vi "KlingerV2 AxisParams.vi"(0 "Axe":u8(ring) items=["W", "X", "Y", "Z"], 1 "TypeMouv":i32(ring) caption="Type de mouvement" items=["Linéaire", "Rotation"], 2 "Nom de l'axe":string, 5 "Type":i32(ring) caption="Type de moteur" items=["UE30", "UE72"], 7 "FactConv":dbl=0.01 caption="Facteur de\nConversion\n(m/pas ou °/pas)", 11 "error in":errorcluster, 12 "Encodeur":bool caption="Possède un\nEncodeur", 13 "MiseàZéro":bool caption="Possède un\nInterrupteur d'origine") -> (4 "Encodeur Out":bool caption="Possède un\nEncodeur", 6 "Nom Out":string, 8 "CorrParams out":T1={"CorrActive"=FALSE, "ErreurLim"=0.1, "NbrEssais"=3} caption="Paramètres de \ncorrection de position" {"NbrEssais" min=1 max=5 step=1; "ErreurLim" min=0.0 max=10.0 step=0.1 format="%#.1f"}, 15 "error out":errorcluster)   [LabVIEW 2019]
doc: "Ce Vi de lire et d'écrire les paramètres des différents axes du fichier .ini"
uses:
  <userlib>/KlingerV2/KlingerV2 Params.ctl
panel:
  in  "CorrParams":T1={"CorrActive"=FALSE, "ErreurLim"=0.1, "NbrEssais"=3} caption="Paramètres de \ncorrection de position" {"NbrEssais" min=1 max=5 step=1; "ErreurLim" min=0.0 max=10.0 step=0.1 format="%#.1f"}
  in  "Id Num":i32 caption="Numéro Id."
  in  "Quitter":bool
  in  "Save":bool
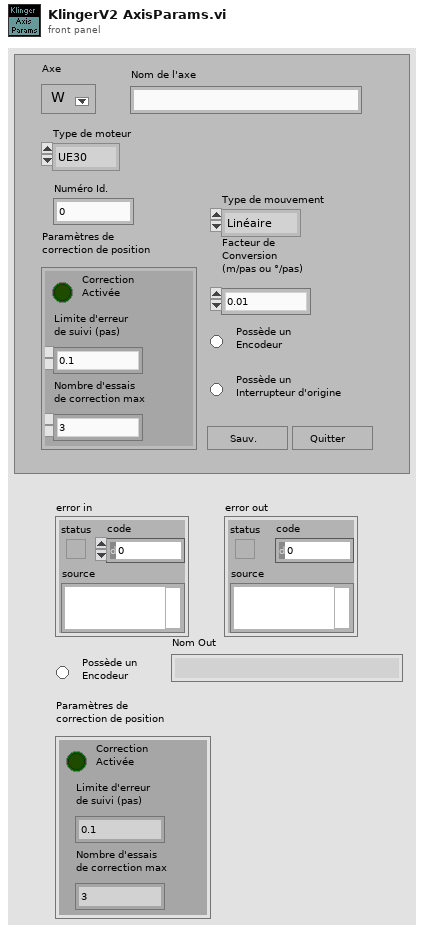
[diagram p1: front panel]
types:
  T1 = cluster{"CorrActive":bool, "ErreurLim":dbl, "NbrEssais":i32}
  T2 = typedef "KlingerV2 Params.ctl" = enum16{"Type", "Origine", "Encodeur", "TypeMouv", "FactConv", "Nom", "CorrParams", "KlingCtrlPar", "Speed", "Acc", "Avance", "Tous"}
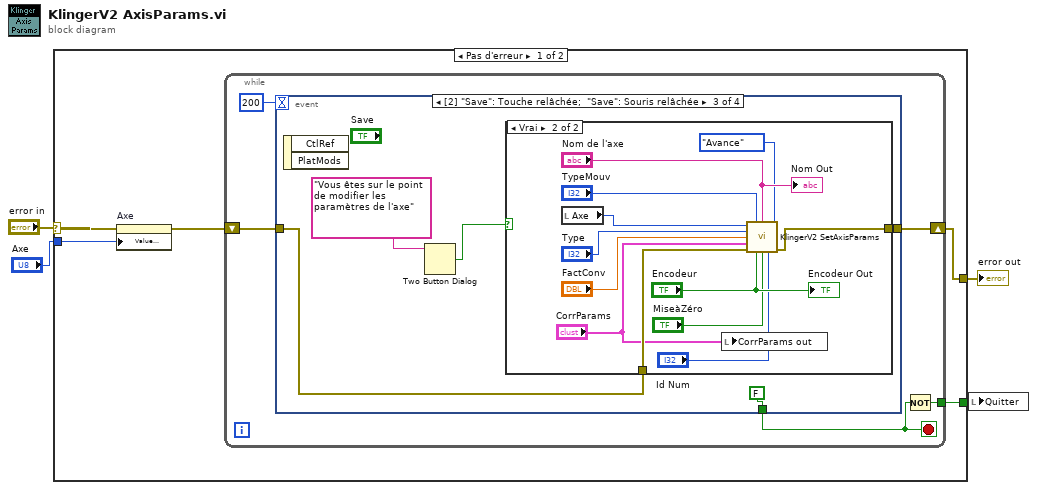
[diagram p0: block diagram]
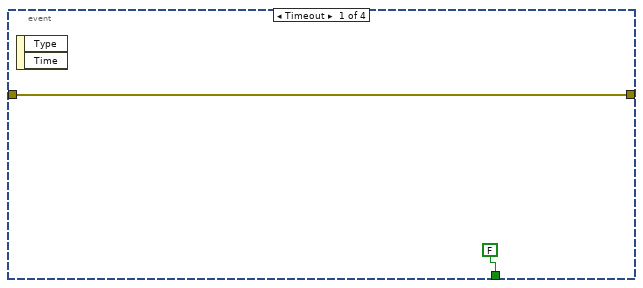
[diagram p2: hidden frame]
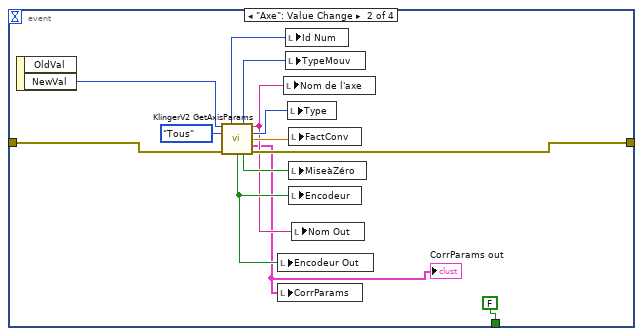
[diagram p3: hidden frame]
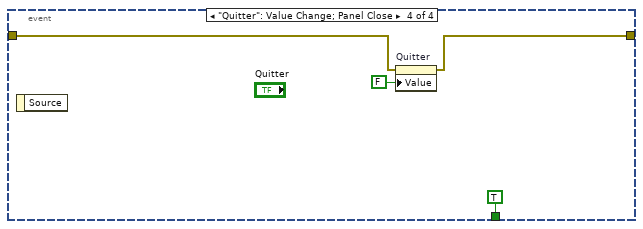
[diagram p5: hidden frame]
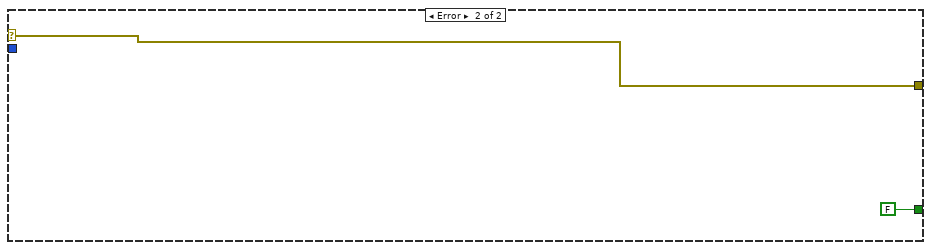
[diagram p6: hidden frame]
diagram:
  n1 = case shown="Pas d'erreur" "error in" {
    selector: "error in" -> [w8 w53]
    tunnel: [w9 w53] -> w4
    tunnel: [w7 FALSE] -> w2
    tunnel: "Axe" -> [w5 _]
    frame No Error {
      n2 = property on="Axe" class="MDér (strict)"(error in=w8, "Value (Signaling)"=w5) -> (error out=w6:errorcluster)  [unwired: 1 in, 1 out]
      n3 = while {
        shift-right: [w12] -> w9
        shift-left: w6 -> [w13]
        tunnel: [w10] -> w7
        stop <- w11 stop-if-true
        n4 = event shown="[2] \"Save\": Touche relâchée;  \"Save\": Souris relâchée" {
          selector: _ -> [_ _ _ _]
          dyn-events: _ -> [_ _ _ _]
          timeout: 200 -> [_ _ _ _]
          tunnel: [FALSE FALSE FALSE TRUE] -> w11
          tunnel: w13 -> [w15 w27 w33 w49]
          tunnel: [w15 w26 w32 w48] -> w12
          event Timeout {
            n5 = event-data() -> ()  [unwired: 1 in, 2 out]
          }
          event "Axe": Value Change {
            n6 = event-data() -> ("NewVal"=w28:u8)  [unwired: 1 in, 1 out]
            n7 = call <userlib>:"KlingerV2 GetAxisParams.vi"("Axe"=w28, "Param"=KlingerV2_Params."Tous", "error in"=w27) -> ("ID Number"=w20:i32, "TypeMouv"=w25:i32, "Nom de l'axe"=w18:string, "Type"=w24:i32, "FactConv"=w23:dbl, "CorrParams"=w17:T1, "Encodeur"=w19:bool, "Origine"=w22:bool, "error out"=w26:errorcluster)  [unwired: 3 in, 1 out]
            "CorrParams out" <- w17
            n8 = local write "Encodeur Out"(w19) -> ()
            n9 = local write "CorrParams"(w17) -> ()
            n10 = local write "Nom de l'axe"(w18) -> ()
            n11 = local write "Id Num"(w20) -> ()
            n12 = local write "TypeMouv"(w25) -> ()
            n13 = local write "Type"(w24) -> ()
            n14 = local write "FactConv"(w23) -> ()
            n15 = local write "MiseàZéro"(w22) -> ()
            n16 = local write "Encodeur"(w19) -> ()
            n17 = local write "Nom Out"(w18) -> ()
          }
          event "Save": Key Up; "Save": Mouse Up {
            n18 = event-data() -> ()  [unwired: 1 in, 2 out]
            n19 = Two Button Dialog(message="Vous êtes sur le point de modifier les paramètres de l'axe") -> (T button?=w30:bool)  [unwired: 2 in]
            n20 = case shown="Vrai" w30 {
              tunnel: w33 -> [w35 w43]
              tunnel: [w35 w42] -> w32
              frame False {
              }
              frame True {
                n21 = local read "Axe"() -> (w39:u8)
                n22 = local write "CorrParams out"("CorrParams") -> ()
                n23 = call <userlib>:"KlingerV2 SetAxisParams.vi"("Axe"=w39, "TypeMouv"="TypeMouv", "Nom de l'axe"="Nom de l'axe", "Param"=KlingerV2_Params."Avance", "Type"="Type", "FactConv"="FactConv", "CorrParams"="CorrParams", "error in"=w43, "Encodeur"="Encodeur", "Origine"="MiseàZéro", "Id Num"="Id Num") -> ("error out"=w42:errorcluster)  [unwired: 4 in]
                "Nom Out" <- "Nom de l'axe"
                "Encodeur Out" <- "Encodeur"
              }
            }
          }
          event "Quitter": Value Change; Panel Close {
            n24 = event-data() -> ()  [unwired: 1 in, 1 out]
            n25 = property on="Quitter" class="Bool (strict)"(error in=w49, "Value"=FALSE ("Quitter")) -> (error out=w48:errorcluster)  [unwired: 1 in, 1 out]
          }
        }
        n26 = Not(x=w11) -> (.not. x?=w10:bool)
      }
    }
    frame Error {
    }
  }
  "error out" <- w4
  n27 = local write "Quitter"(w2) -> ()
